vi "Tiny_ReadDebugScript.vi"(3 "read buffer":string) -> (1 "read buffer":string)   [LabVIEW 2014]
panel:
  out "Numeric":i32
  out "Vars":string[](array[string])
  out "array":string[](array[string])
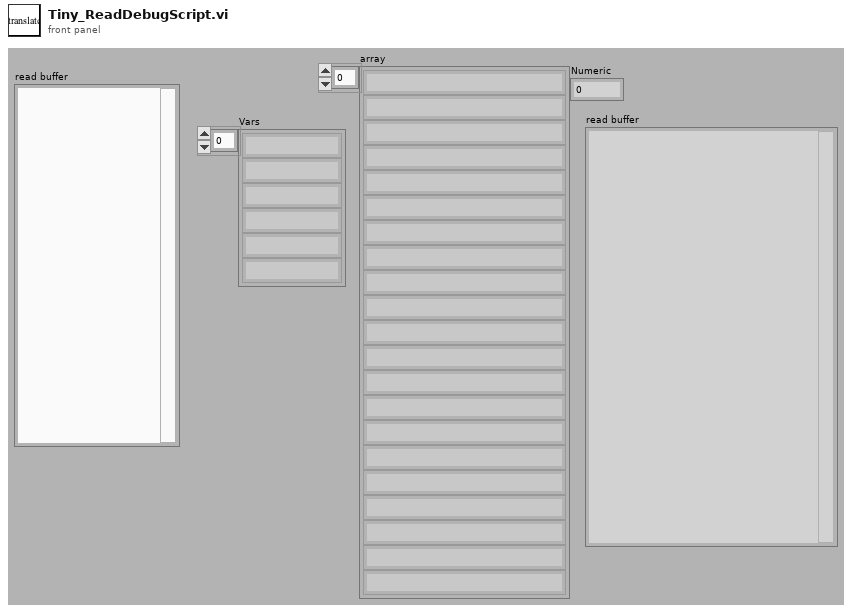
[diagram p1: front panel]
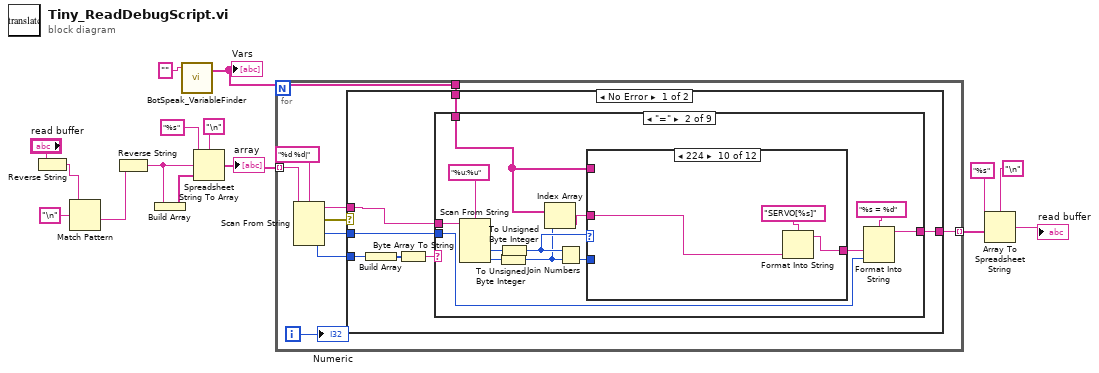
[diagram p0: block diagram]
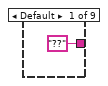
[diagram p2: hidden frame]
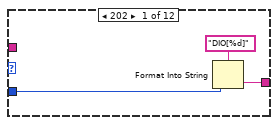
[diagram p3: hidden frame]
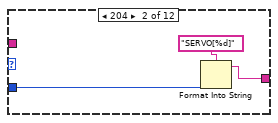
[diagram p4: hidden frame]
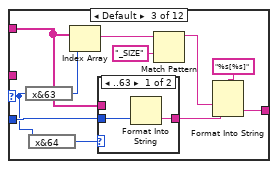
[diagram p5: hidden frame]
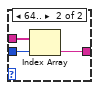
[diagram p6: hidden frame]
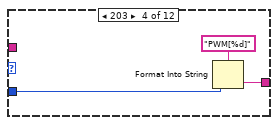
[diagram p7: hidden frame]
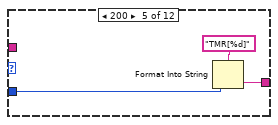
[diagram p8: hidden frame]
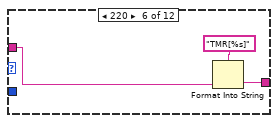
[diagram p9: hidden frame]
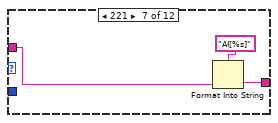
[diagram p10: hidden frame]
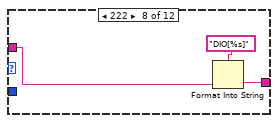
[diagram p11: hidden frame]
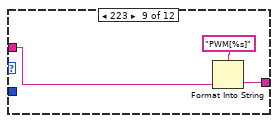
[diagram p12: hidden frame]
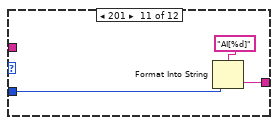
[diagram p13: hidden frame]
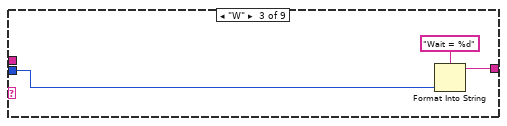
[diagram p15: hidden frame]
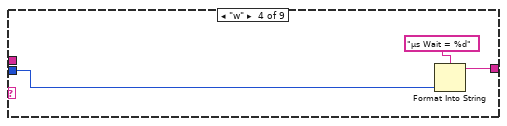
[diagram p16: hidden frame]
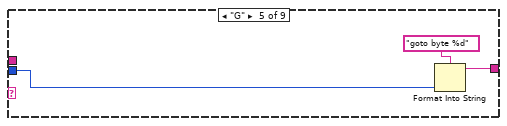
[diagram p17: hidden frame]
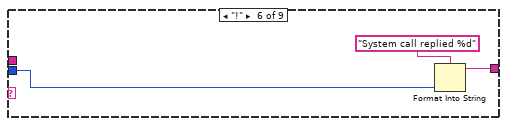
[diagram p18: hidden frame]
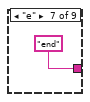
[diagram p19: hidden frame]
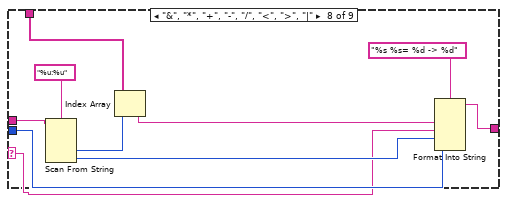
[diagram p20: hidden frame]
diagram:
  n1 = Reverse String(1:"read buffer") -> (0:w3:string)
  n2 = Match Pattern(string=w3, regular expression="\n") -> (after substring=w1:string)  [unwired: 1 in, 3 out]
  n3 = Reverse String(1:w1) -> (0:w2:string)
  n4 = Build Array(w2) -> (w15:string[])
  n5 = call <userlib>:"BotSpeak_VariableFinder.vi"("variable name"="") -> ("Variables"=w11:string[])  [unwired: 2 in, 1 out]
  "Vars" <- w11
  n6 = Spreadsheet String To Array(delimiter (Tab)="\n", format string="%s", spreadsheet string=w2, array type (2D Dbl)=w15) -> (array=w10:string[])
  "array" <- w10
  n7 = for {
    tunnel: w10 -> [w22] mode=indexing
    tunnel: w11 -> [w24]
    tunnel: [w23] -> w6 mode=indexing
    i -> [w16]
    n8 = Scan From String(format string="%d %d|", input string=w22) -> (remaining string=w20:string, error out=w18:errorcluster, output 1=w19:i32, output 2=w17:i32)  [unwired: 4 in, 1 out]
    n9 = case shown="No Error" w18 {
      tunnel: w24 -> [w31 _]
      tunnel: [w30 w125] -> w23
      tunnel: w20 -> [w26 w125]
      tunnel: w19 -> [w25 _]
      tunnel: w17 -> [w29 _]
      frame No Error {
        n10 = Build Array(w29) -> (w28:i32[])
        n11 = Byte Array To String(unsigned byte array=w28) -> (string=w27:string)
        n12 = case shown="\"=\"" w27 {
          selector: w27 -> [_ _ _ _ _ _ _ w105 _]
          tunnel: w31 -> [_ w34 _ _ _ _ _ w111 _]
          tunnel: ["??" w44 w94 w97 w100 w103 "end" ("format string") w114 w124] -> w30
          tunnel: w26 -> [_ w43 _ _ _ _ _ w109 w121]
          tunnel: w25 -> [_ w37 w92 w95 w98 w101 _ w113 w117]
          frame Default {
          }
          frame "=" {
            n13 = Scan From String(format string="%u:%u", input string=w43) -> (output 1=w39:u32, output 2=w38:u32)  [unwired: 4 in, 3 out]
            n14 = To Unsigned Byte Integer(number=w38) -> (unsigned 8bit integer=w33:u8)
            n15 = To Unsigned Byte Integer(number=w39) -> (unsigned 8bit integer=w36:u8)
            n16 = Index Array(array=w34, index=w33) -> (element=w35:string)
            n17 = Join Numbers(hi=w36, lo=w33) -> ()  [unwired: 1 out]
            n18 = case shown="224" w36 {
              selector: w36 -> [_ _ w52 _ _ _ _ _ _ _ _ _]
              tunnel: [w45 w49 w60 w67 w70 w74 w77 w80 w83 w85 w88 w91] -> w40
              tunnel: w33 -> [w46 w48 w53 w68 w71 _ _ _ _ _ w89 _]
              tunnel: w35 -> [_ _ _ _ _ w73 w76 w79 w82 w86 _ w91]
              tunnel: w34 -> [_ _ w55 _ _ _ _ _ _ _ _ _]
              frame 202 {
                n19 = Format Into String(format string="DIO[%d]", w46) -> (resulting string=w45:string)  [unwired: 2 in, 1 out]
              }
              frame 204 {
                n20 = Format Into String(format string="SERVO[%d]", w48) -> (resulting string=w49:string)  [unwired: 2 in, 1 out]
              }
              frame Default {
                n21 = expression code="x&63"(w52) -> (w58:u8)
                n22 = expression code="x&64"(w52) -> (w51:u8)
                n23 = Index Array(array=w55, index=w58) -> (element=w57:string)
                n24 = case shown="..63" w51 {
                  tunnel: w55 -> [_ w66]
                  tunnel: [w62 w65] -> w54
                  tunnel: w53 -> [w63 w64]
                  frame ..63 {
                    n25 = Format Into String(w63) -> (resulting string=w62:string)  [unwired: 3 in, 1 out]
                  }
                  frame 64.. {
                    n26 = Index Array(array=w66, index=w64) -> (element=w65:string)
                  }
                }
                n27 = Match Pattern(string=w57, regular expression="_SIZE") -> (before substring=w59:string)  [unwired: 1 in, 3 out]
                n28 = Format Into String(format string="%s[%s]", w59, w54) -> (resulting string=w60:string)  [unwired: 2 in, 1 out]
              }
              frame 203 {
                n29 = Format Into String(format string="PWM[%d]", w68) -> (resulting string=w67:string)  [unwired: 2 in, 1 out]
              }
              frame 200 {
                n30 = Format Into String(format string="TMR[%d]", w71) -> (resulting string=w70:string)  [unwired: 2 in, 1 out]
              }
              frame 220 {
                n31 = Format Into String(format string="TMR[%s]", w73) -> (resulting string=w74:string)  [unwired: 2 in, 1 out]
              }
              frame 221 {
                n32 = Format Into String(format string="AI[%s]", w76) -> (resulting string=w77:string)  [unwired: 2 in, 1 out]
              }
              frame 222 {
                n33 = Format Into String(format string="DIO[%s]", w79) -> (resulting string=w80:string)  [unwired: 2 in, 1 out]
              }
              frame 223 {
                n34 = Format Into String(format string="PWM[%s]", w82) -> (resulting string=w83:string)  [unwired: 2 in, 1 out]
              }
              frame 224 {
                n35 = Format Into String(format string="SERVO[%s]", w86) -> (resulting string=w85:string)  [unwired: 2 in, 1 out]
              }
              frame 201 {
                n36 = Format Into String(format string="AI[%d]", w89) -> (resulting string=w88:string)  [unwired: 2 in, 1 out]
              }
              frame ..127 {
              }
            }
            n37 = Format Into String(format string="%s = %d", w40, w37) -> (resulting string=w44:string)  [unwired: 2 in, 1 out]
          }
          frame "W" {
            n38 = Format Into String(format string="Wait = %d", w92) -> (resulting string=w94:string)  [unwired: 2 in, 1 out]
          }
          frame "w" {
            n39 = Format Into String(format string="µs Wait = %d", w95) -> (resulting string=w97:string)  [unwired: 2 in, 1 out]
          }
          frame "G" {
            n40 = Format Into String(format string="goto byte %d", w98) -> (resulting string=w100:string)  [unwired: 2 in, 1 out]
          }
          frame "!" {
            n41 = Format Into String(format string="System call replied %d", w101) -> (resulting string=w103:string)  [unwired: 2 in, 1 out]
          }
          frame "e" {
          }
          frame "&", "*", "+", "-", "/", "<", ">", "|" {
            n42 = Scan From String(format string="%u:%u", input string=w109) -> (output 1=w108:u32, output 2=w107:u32)  [unwired: 4 in, 3 out]
            n43 = Index Array(array=w111, index=w108) -> (element=w106:string)
            n44 = Format Into String(format string="%s %s= %d -> %d", w106, w105, w107, w113) -> (resulting string=w114:string)  [unwired: 2 in, 1 out]
          }
          frame "I", "i" {
            n45 = Scan From String(format string="(%u %u %u)", input string=w121) -> (output 1=w115:u32, output 2=w116:u32, output 3=w118:u32)  [unwired: 5 in, 3 out]
            n46 = Build Array(w116) -> (w120:u32[])
            n47 = Byte Array To String(unsigned byte array=w120) -> (string=w119:string)
            n48 = Format Into String(format string="If (%d %s %d) -> %d", w115, w119, w118, w117) -> (resulting string=w124:string)  [unwired: 2 in, 1 out]
          }
        }
      }
      frame Error {
      }
    }
    "Numeric" <- w16
  }
  n49 = Array To Spreadsheet String(delimiter (Tab)="\n", array=w6, 3:"%s" ("format string")) -> (spreadsheet string=→"read buffer":string)
